vi "Set 2D Array Double.vi"(5 "use temporary file? (F)":bool, 8 "error in":errorcluster, 9 "value":dbl[][](array[numeric]), 10 "variable name":string, 11 "GOLPI ref. in":T1={"pipe handle"={"lv_proc.dll file path"=path "", "process instance handle"=[], "debug mode"=FALSE, "debug data"=[]}, "fast read timeout [ms]"=500, "fast read settle time [ms]"=10, "fast read to multiple [ms]"=1, "max elements per input line"=100, "slow read timeout [ms]"=5000, "stdin double format specifier"="%_16e", "max elements per stdout output column"=100}) -> (0 "error out":errorcluster, 3 "GOLPI ref. out":T1={"pipe handle"={"lv_proc.dll file path"=path "", "process instance handle"=[], "debug mode"=FALSE, "debug data"=[]}, "fast read timeout [ms]"=500, "fast read settle time [ms]"=10, "fast read to multiple [ms]"=1, "max elements per input line"=100, "slow read timeout [ms]"=5000, "stdin double format specifier"="%_16e", "max elements per stdout output column"=100})   [LabVIEW 2013, in "GOLPI library.lvlib"]
doc: "Part of polymorph Set Variable.vi"
uses:
  GOLPI library.lvlib
  Public/GOLPI reference Type Def.ctl
  LV Process source distribution/Pipe Handle.ctl
  LV Process source distribution/LV Process library.lvlib
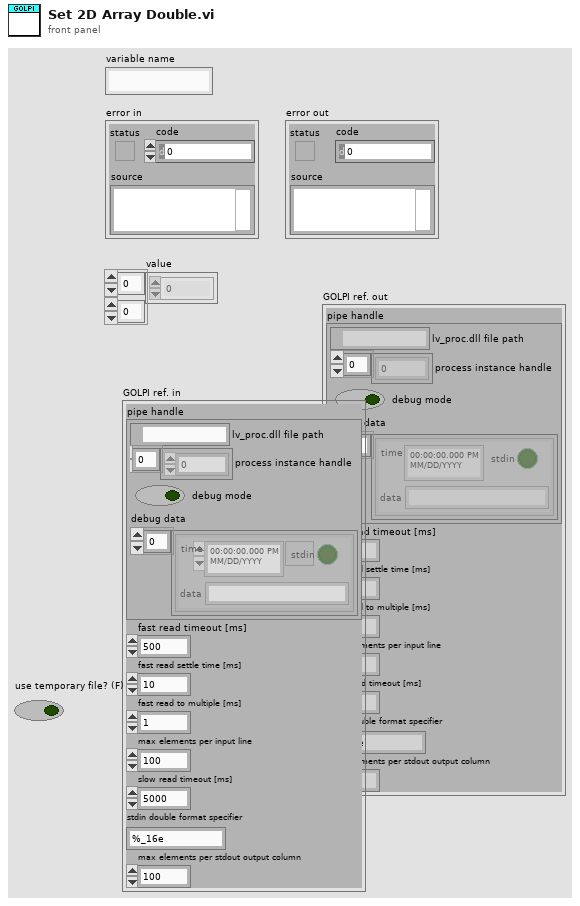
[diagram p1: front panel]
types:
  T1 = typedef "GOLPI library.lvlib/GOLPI reference Type Def.ctl" = cluster{"pipe handle":T2, "fast read timeout [ms]":u32, "fast read settle time [ms]":u32, "fast read to multiple [ms]":u32, "max elements per input line":u32, "slow read timeout [ms]":u32, "stdin double format specifier":string, "max elements per stdout output column":u32}
  T2 = typedef "LV Process library.lvlib/Pipe Handle.ctl" = cluster{"lv_proc.dll file path":path, "process instance handle":u32[], "debug mode":bool, "debug data":cluster{"time":timestamp, "stdin":bool, "data":string}[]}
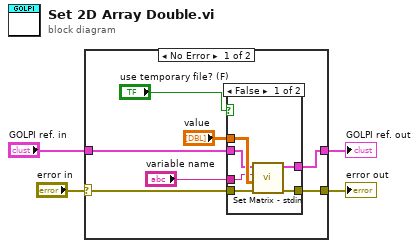
[diagram p0: block diagram]
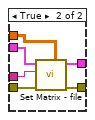
[diagram p2: hidden frame]
diagram:
  n1 = case shown="No Error" "error in" {
    selector: "error in" -> [w9 w25]
    tunnel: [w8 w25] -> w4
    tunnel: "GOLPI ref. in" -> [w7 w24]
    tunnel: [w6 w24] -> w1
    frame No Error {
      n2 = case shown="False" "use temporary file? (F)" {
        tunnel: "value" -> [w17 w18]
        tunnel: "variable name" -> [w16 w19]
        tunnel: w9 -> [w15 w23]
        tunnel: [w14 w22] -> w8
        tunnel: w7 -> [w13 w20]
        tunnel: [w12 w21] -> w6
        frame False {
          n3 = call "Set Matrix - stdin.vi"("error in"=w15, "value"=w17, "variable name"=w16, "GOLPI ref. in"=w13) -> ("error out"=w14:errorcluster, "GOLPI ref. out"=w12:T1)  [unwired: 6 in]
        }
        frame True {
          n4 = call "Set Matrix - file.vi"("double array"=w18, "error in (no error)"=w23, "variable name"=w19, "GOLPI ref. in"=w20) -> ("error out"=w22:errorcluster, "GOLPI ref. out"=w21:T1)  [unwired: 6 in]
        }
      }
    }
    frame Error {
    }
  }
  "error out" <- w4
  "GOLPI ref. out" <- w1
